vi "9224_UI.vi"(8 "error in (no error)":errorcluster, 11 "Node Ptr":T2 format="%.0x") -> (0 "error out":errorcluster)   [LabVIEW 2019, in "Modules.lvlib" / "9224.lvclass"]
uses:
  9224.lvclass
  <vilib>/NI VeriStand/Custom Device API/Custom Device Item Ref.ctl
  RSI Module/SubPanel Command.ctl
  Conversion Time.ctl
  C:/Users/nitest/Desktop/Git 2019/niveristand-scan-engine-module-libraries/Source/RSI Module/RSI Module.lvclass
  9224.lvclass/9224.ctl
  RSI Module/RSI Module.lvclass
  <vilib>/NI VeriStand/Custom Device API/Custom Device API.lvlib
panel:
  in  "Conversion Time":T1 items=["High Speed (1k S/s)", "Medium Speed (100 S/s)", "Medium Resolution (50/60Hz Rejection - 12 S/s)", "High Resolution (50/60Hz rejection - 2 S/s)"]
  in  "SubPanel Event":refnum<user-event>
  in  "Header":cluster{"Section Name":string}={"Section Name"="NI 9205 Settings"}
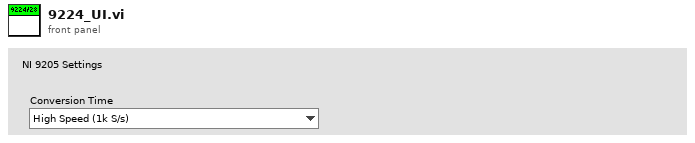
[diagram p1: front panel]
types:
  T1 = typedef "Modules.lvlib/9224.lvclass/Conversion Time.ctl" = u16
  T2 = typedef "Custom Device API.lvlib/Custom Device Item Ref.ctl" = u64
  T3 = typedef "Modules.lvlib/RSI Module.lvclass/Module Models.ctl" = enum16{"Empty", "NI 9201", "NI 9203", "NI 9205", "NI 9206", "NI 9207", "NI 9208", "NI 9209", "NI 9210", "NI 9211", "NI 9212", "NI 9213", "NI 9214", "NI 9215", "NI 9216", "NI 9217", "NI 9219", "NI 9220", "NI 9221", "NI 9222", "NI 9223", "NI 9224", "NI 9225", "NI 9226", "NI 9227", "NI 9228", "NI 9229", "NI 9233", "NI 9234", "NI 9235", "NI 9236", "NI 9237", "NI 9239", "NI 9242", "NI 9244", "NI 9253", "NI 9263", "NI 9264", "NI 9265", "NI 9266", "NI 9269", "NI 9344", "NI 9350", "NI 9375", "NI 9401", "NI 9402", "NI 9403", "NI 9411", "NI 9421", "NI 9422", "NI 9423", "NI 9425", "NI 9426", "NI 9435", "NI 9436", "NI 9437", "NI 9472", "NI 9474", "NI 9475", "NI 9476", "NI 9477", "NI 9478", "NI 9481", "NI 9482", "NI 9485"}
  T4 = typedef "Modules.lvlib/RSI Module.lvclass/SubPanel Command.ctl" = enum16{"Stop"}
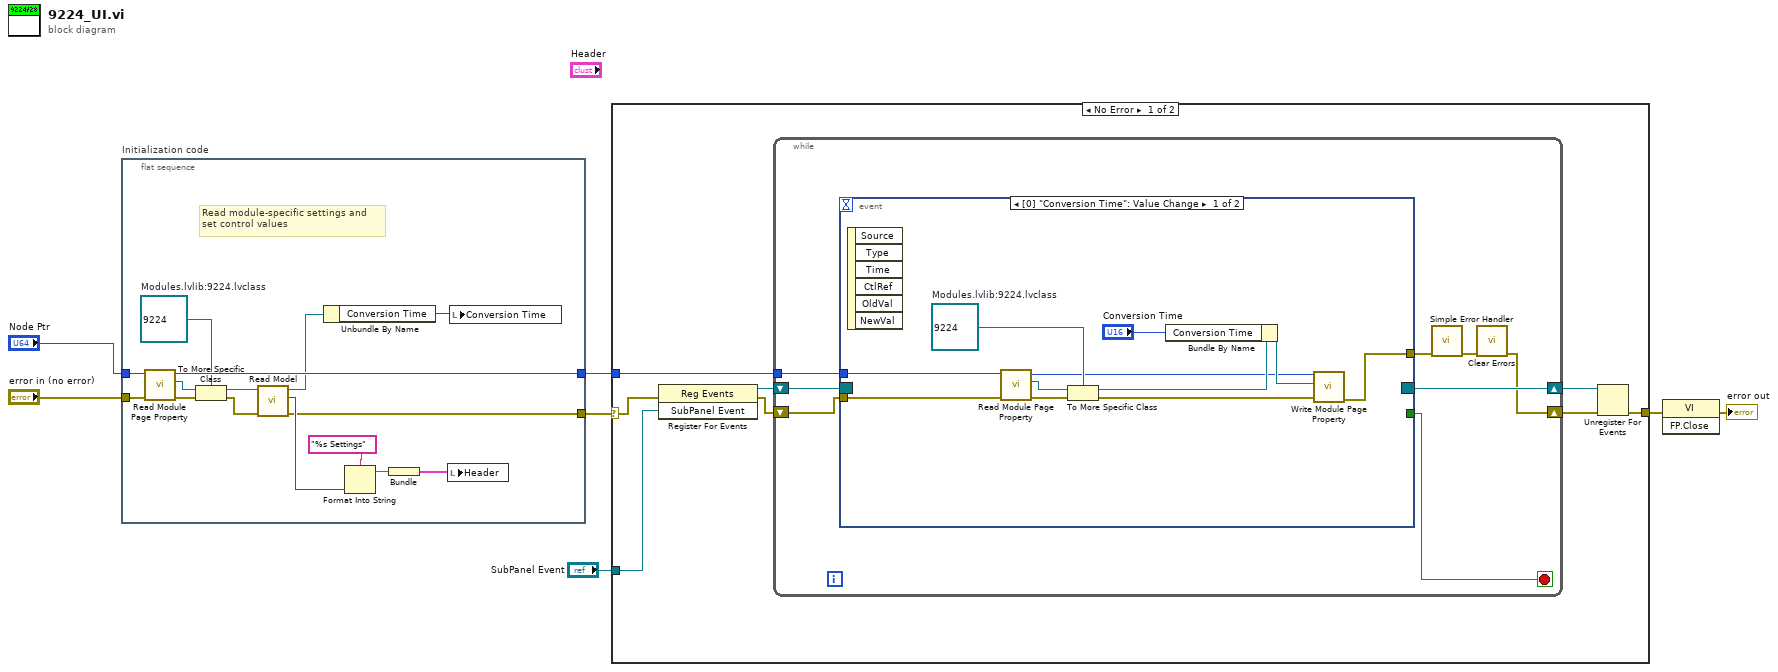
[diagram p0: block diagram]
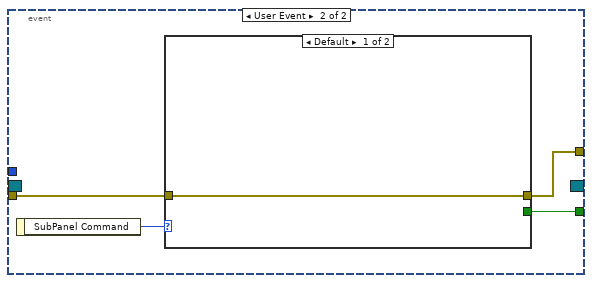
[diagram p2: hidden frame]
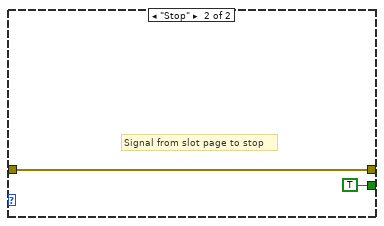
[diagram p3: hidden frame]
diagram:
  n1 = flat-sequence "Initialization code" {
    tunnel: [w22] -> w4
    tunnel: "error in (no error)" -> [w13]
    tunnel: [w12] -> w6
    tunnel: "Node Ptr" -> [w11]
    frame #0 {
      w14 = refnum<class "9224.lvclass"> refnum  # Modules.lvlib:9224.lvclass
      # "Read module-specific settings and\nset control values"
      n2 = call "Read Module Page Property.vi"("error in (no error)"=w13, "Node Ptr In"=w11) -> ("error out"=w21:errorcluster, "RSI Module"=w20:refnum<class "RSI Module.lvclass">, "Node Ptr Out"=w22:T2)  [unwired: 7 in]
      n3 = To More Specific Class(target class=w14, reference=w20, error in=w21) -> (specific class reference=w15:refnum<class "9224.lvclass">, error out=w19:errorcluster)
      n4 = call "Read Model.vi"("error in (no error)"=w19, "RSI Module in"=w15) -> ("error out"=w12:errorcluster, "Model"=w18:T3, "RSI Module out"=w10:refnum<class "9224.lvclass">)  [unwired: 7 in]
      n5 = Unbundle By Name(w10) -> ("Conversion Time"=w9:T1)
      n6 = Format Into String(format string="%s Settings", w18) -> (resulting string=w16:string)  [unwired: 2 in, 1 out]
      n7 = Bundle(w16) -> (w8:cluster{string})  [unwired: 1 in]
      n8 = local write "Header"(w8) -> ()
      n9 = local write "Conversion Time"(w9) -> ()
    }
  }
  n10 = case shown="No Error" w6 {
    selector: w6 -> [w30 w57]
    tunnel: "SubPanel Event" -> [w29 _]
    tunnel: w4 -> [w27 _]
    tunnel: [w23 w57] -> w2
    frame No Error {
      n11 = register-events(error in=w30, w29) -> (reference out=w26:refnum<event-registration>, error out=w28:errorcluster)  [unwired: 1 in]
      n12 = while {
        tunnel: w27 -> [w37]
        shift-right: [w32] -> w24
        shift-left: w26 -> [w36]
        shift-right: [w31] -> w25
        shift-left: w28 -> [w38]
        stop <- w35 stop-if-true
        n13 = event shown="[0] \"Conversion Time\": Value Change" {
          selector: w36 -> [_ _]
          dyn-events: [_ _] -> w32
          timeout: _ -> [_ _]
          tunnel: w38 -> [w48 w52]
          tunnel: w37 -> [w42 _]
          tunnel: [_ w51] -> w35
          tunnel: [w40 w50] -> w33
          event Value Change {
            w47 = refnum<class "9224.lvclass"> refnum  # Modules.lvlib:9224.lvclass
            n14 = event-data() -> ()  [unwired: 1 in, 6 out]
            n15 = call "Read Module Page Property.vi"("error in (no error)"=w48, "Node Ptr In"=w42) -> ("error out"=w49:errorcluster, "RSI Module"=w46:refnum<class "RSI Module.lvclass">, "Node Ptr Out"=w39:T2)  [unwired: 7 in]
            n16 = To More Specific Class(target class=w47, reference=w46, error in=w49) -> (specific class reference=w44:refnum<class "9224.lvclass">, error out=w45:errorcluster)
            n17 = Bundle By Name(cluster=w44, "Conversion Time"="Conversion Time") -> (w43:refnum<class "9224.lvclass">)
            n18 = call "Write Module Page Property.vi"("error in (no error)"=w45, "RSI Module"=w43, "Node Ptr In"=w39) -> ("error out"=w40:errorcluster)  [unwired: 6 in, 2 out]
          }
          event User Event {
            n19 = event-data() -> ("SubPanel Command"=w53:T4)  [unwired: 1 in]
            n20 = case shown="Default" w53 {
              tunnel: w52 -> [w54 w55]
              tunnel: [w54 w55] -> w50
              tunnel: [_ TRUE] -> w51
              frame Default {
              }
              frame "Stop" {
                # "Signal from slot page to stop"
              }
            }
          }
        }
        n21 = call <vilib>:"Simple Error Handler.vi"("error in (no error)"=w33) -> ("error out"=w34:errorcluster)  [unwired: 1 in, 7 out]
        n22 = call <vilib>:"Clear Errors.vi"("error in (no error)"=w34) -> ("error out"=w31:errorcluster)  [unwired: 1 in, 5 out]
      }
      n23 = Unregister For Events(event registration refnum=w24, error in=w25) -> (error out=w23:errorcluster)
    }
    frame Error {
    }
  }
  n24 = invoke class="VI" method="FP.Close"(error in=w2) -> (error out=→"error out":errorcluster)  [unwired: 2 in, 2 out]
